vi "Calc Init.vi"(8 "error in (no error)":errorcluster, 10 "Config":refnum<class "Channel Config.lvclass">, 11 "Max Calc in":refnum<class "Max Calc.lvclass">) -> (0 "error out":errorcluster, 3 "Max Calc out":refnum<class "Max Calc.lvclass">)   [LabVIEW 2020, in "VolatusCalcs.lvlib" / "Max Calc.lvclass"]
uses:
  Max Calc.lvclass
  Max Calc.lvclass/Max Calc.ctl
  VolatusConfig/VolatusConfigElement/VolatusConfigElement.lvclass
  lv-cdm/CDM-Config/Config Element/Config Element.lvclass
  VolatusConfig/Channel/Channel Config.lvclass
  C:/dev/lv20CE/relink/lv-volatus/VolatusConfig/VolatusConfigElement/VolatusConfigElement.lvclass
  C:/dev/lv20CE/relink/lv-volatus/VolatusConfig/Channel/Channel Config.lvclass
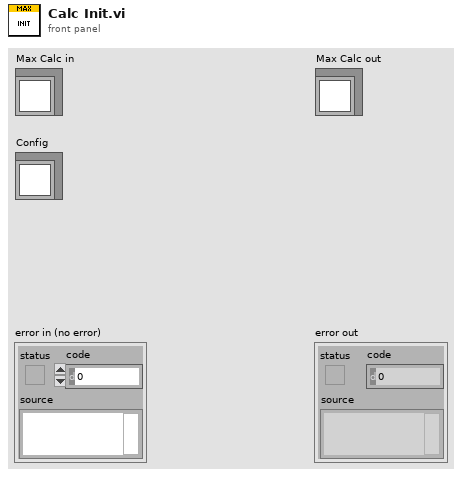
[diagram p1: front panel]
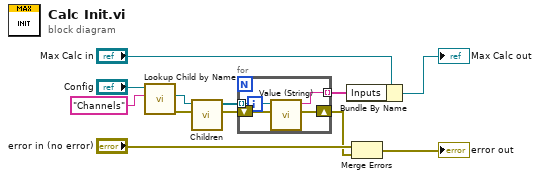
[diagram p0: block diagram]
diagram:
  n1 = call "Lookup Child by Name.vi"("Child Name"="Channels", "VolatusConfigElement in"="Config") -> ("error out"=w8:errorcluster, "Child"=w7:refnum<class "Config Element.lvclass">)  [unwired: 6 in, 2 out]
  n2 = call "Children.vi"("error in (no error)"=w8, "Config Element in"=w7) -> ("error out"=w6:errorcluster, "Elements"=w5:refnum<class "Config Element.lvclass">[])  [unwired: 8 in]
  n3 = for {
    shift-right: [w14] -> w1
    shift-left: w6 -> [w16]
    tunnel: w5 -> [w15] mode=indexing
    tunnel: [w13] -> w3 mode=indexing
    n4 = call "Value (String).vi"("error in (no error)"=w16, "Config Element in"=w15) -> ("error out"=w14:errorcluster, "String Value"=w13:string)  [unwired: 8 in]
  }
  n5 = Bundle By Name(cluster="Max Calc in", "Inputs"=w3) -> (→"Max Calc out":refnum<class "Max Calc.lvclass">)
  n6 = Merge Errors("error in (no error)", w1) -> (→"error out":errorcluster)
